vi "To String (String).vi"(8 "error in (no error)":errorcluster, 11 "JSON Value in":variant) -> (0 "error out":errorcluster, 3 "String":string)   [LabVIEW 2017, in "Advanced Variant Tools.lvlib"]
doc: "Flattens the given JSON data to a string."
uses:
  Advanced Variant Tools.lvlib
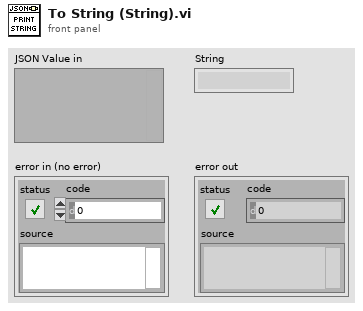
[diagram p1: front panel]
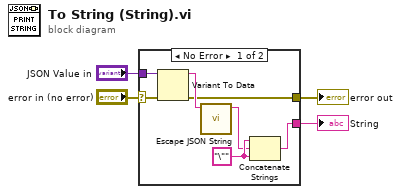
[diagram p0: block diagram]
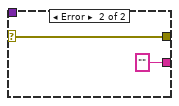
[diagram p2: hidden frame]
diagram:
  n1 = case shown="No Error" "error in (no error)" {
    selector: "error in (no error)" -> [w6 w12]
    tunnel: "JSON Value in" -> [w8 _]
    tunnel: [w10 ""] -> w3
    tunnel: [w5 w12] -> w2
    frame No Error {
      w11 = "\"" ("string")
      n2 = Variant To Data(error in=w6, Variant=w8) -> (data=w7:string, error out=w5:errorcluster)  [unwired: 1 in]
      n3 = call "Escape JSON String.vi"("value"=w7) -> ("escaped string"=w9:string)  [unwired: 10 in]
      n4 = Concatenate Strings(w11, w9, w11) -> (w10:string)
    }
    frame Error {
    }
  }
  "String" <- w3
  "error out" <- w2
